vi "test FIFOs.vi"(8 "error in (no error)":errorcluster, 11 "TestCase in":refnum<class "Configuration Tests.lvclass">) -> (0 "error out":errorcluster, 3 "TestCase out":refnum<class "Configuration Tests.lvclass">)   [LabVIEW 2017, in "Configuration Tests.lvclass"]
uses:
  Configuration Tests.lvclass
  Engine/Classes/Transfer Group/Transfer Group.lvclass
  Engine/Classes/Transfer Group/Transfer Group.lvclass/Transfer Group.ctl
  Engine/Classes/Timing/Timing.lvclass/Timing.ctl
  Engine/Classes/Debug/Debug Flags/Debug Flags.lvclass/Debug Flags.ctl
  Engine/Classes/Debug/FIFO Flags/FIFO Flags.lvclass/FIFO Flags.ctl
  Engine/Classes/Transfer Group/Get Return FIFO.vi
  Engine/Classes/Transfer Group/Get Timing.vi
  Engine/Classes/Timing/Get Iteration.vi
  Engine/Classes/Transfer Group/Get Debug Flags.vi
  Engine/Classes/Debug/Debug Flags/Get FIFO Flags.vi
  Engine/Classes/Debug/FIFO Flags/Get Infinite Timeouts.vi
  Engine/Classes/Transfer Group/Errors.vi
  Engine/Classes/Transfer Group/Return Timeout Error.vi
  <vilib>/addons/_JKI Toolkits/VI Tester/TestCase.llb/TestCase.lvclass
  C:/Program Files (x86)/National Instruments/LabVIEW 2017/vi.lib/addons/_JKI Toolkits/VI Tester/TestCase.llb/TestCase.lvclass
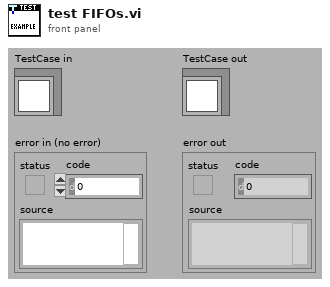
[diagram p1: front panel]
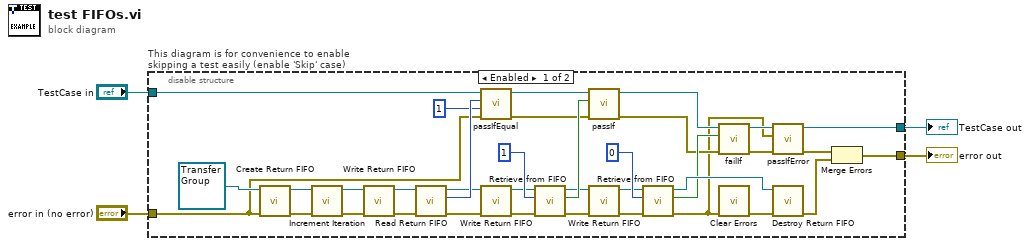
[diagram p0: block diagram]
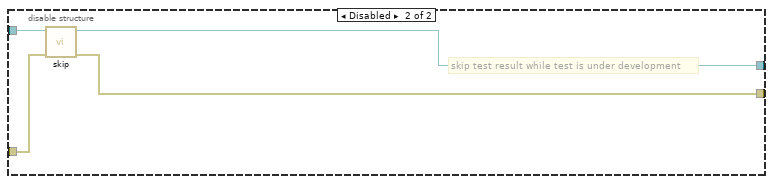
[diagram p2: hidden frame]
diagram:
  n1 = disable-structure "This diagram is for convenience to enable skipping a test easily (enable 'Skip' case)" shown="Enabled" {
    disable-tunnel: "TestCase in" -> [w33 w44]
    disable-tunnel: [w7 w42] -> w1
    disable-tunnel: [w17 w43] -> w3
    disable-tunnel: "error in (no error)" -> [w25 w41]
    frame Enabled {
      n2 = call "Create Return FIFO.vi"("error in (no error)"=w25, "Transfer Group in"=refnum<class "Transfer Group.lvclass"> refnum) -> ("error out"=w40:errorcluster, "Transfer Group out"=w35:refnum<class "Transfer Group.lvclass">)  [unwired: 8 in]
      n3 = call "Increment Iteration.vi"("error in (no error)"=w40, "Transfer Group in"=w35) -> ("error out"=w36:errorcluster, "Transfer Group out"=w34:refnum<class "Transfer Group.lvclass">)  [unwired: 8 in]
      n4 = call "Write Return FIFO.vi"("error in (no error)"=w36, "Transfer Group in"=w34) -> ("error out"=w38:errorcluster, "Transfer Group out"=w39:refnum<class "Transfer Group.lvclass">)  [unwired: 7 in, 1 out]
      n5 = call "Read Return FIFO.vi"("error in (no error)"=w38, "Transfer Group in"=w39) -> ("error out"=w26:errorcluster, "Transfer Group iteration"=w31:u64, "Transfer Group out"=w15:refnum<class "Transfer Group.lvclass">)  [unwired: 6 in, 1 out]
      n6 = call-dynamic "passIfEqual.vi"("error in (no error)"=w25, "y"=u64 1 ("Transfer Group iteration"), "x"=w31, "TestCase in"=w33) -> ("error out"=w18:errorcluster, "TestCase out"=w32:refnum<class "Configuration Tests.lvclass">)  [unwired: 6 in]
      n7 = call "Write Return FIFO.vi"("error in (no error)"=w26, "Transfer Group in"=w15) -> ("error out"=w16:errorcluster, "Transfer Group out"=w14:refnum<class "Transfer Group.lvclass">)  [unwired: 7 in, 1 out]
      n8 = call "Retrieve from FIFO.vi"("error in (no error)"=w16, "expected iteration"=u64 1, "Transfer Group in"=w14) -> ("error out"=w29:errorcluster, "iteration valid?"=w23:bool, "Transfer Group out"=w12:refnum<class "Transfer Group.lvclass">)  [unwired: 6 in]
      n9 = call-dynamic "passIf.vi"("error in (no error)"=w18, "pass"=w23, "TestCase in"=w32) -> ("error out"=w19:errorcluster, "TestCase out"=w24:refnum<class "Configuration Tests.lvclass">)  [unwired: 7 in]
      n10 = call "Write Return FIFO.vi"("error in (no error)"=w29, "Transfer Group in"=w12) -> ("error out"=w13:errorcluster, "Transfer Group out"=w11:refnum<class "Transfer Group.lvclass">)  [unwired: 7 in, 1 out]
      n11 = call "Retrieve from FIFO.vi"("error in (no error)"=w13, "expected iteration"=u64 0, "Transfer Group in"=w11) -> ("error out"=w5:errorcluster, "iteration valid?"=w21:bool, "Transfer Group out"=w22:refnum<class "Transfer Group.lvclass">)  [unwired: 6 in]
      n12 = call-dynamic "failIf.vi"("error in (no error)"=w19, "fail"=w21, "TestCase in"=w24) -> ("error out"=w6:errorcluster, "TestCase out"=w8:refnum<class "Configuration Tests.lvclass">)  [unwired: 7 in]
      n13 = call <vilib>:"Clear Errors.vi"("error in (no error)"=w5) -> ("error out"=w10:errorcluster)  [unwired: 5 in, 1 out]
      n14 = call-dynamic "passIfError.vi"("error in (no error)"=w6, "error"=w5, "TestCase in"=w8) -> ("error out"=w9:errorcluster, "TestCase out"=w7:refnum<class "Configuration Tests.lvclass">)  [unwired: 7 in]
      n15 = call "Destroy Return FIFO.vi"("error in (no error)"=w10, "Transfer Group in"=w22) -> ("error out"=w27:errorcluster)  [unwired: 8 in, 1 out]
      n16 = Merge Errors(w9, w27) -> (w17:errorcluster)
    }
    frame Disabled {
      # "skip test result while test is under development"
      n17 = call <vilib>:"skip.vi"("error in (no error)"=w41, "TestCase in"=w44) -> ("error out"=w43:errorcluster, "TestCase out"=w42:refnum<class "Configuration Tests.lvclass">)  [unwired: 8 in]
    }
  }
  "error out" <- w3
  "TestCase out" <- w1
